vi "Clear All.vi"(8 "error in":errorcluster, 11 "MLTFNC in":refnum<class "MLTFNC.lvclass">) -> (0 "error out":errorcluster, 3 "MLTFNC out":refnum<class "MLTFNC.lvclass">)   [LabVIEW 2019, in "MLTFNC.lvlib" / "MLTFNC.lvclass"]
uses:
  Library/MLTFNC.lvclass
  C:/Users/Public/Documents/Development/builds/Instruments/Instruments.lvlibp/Library/Instruments.lvclass
  Library/MLTFNC.lvclass/MLTFNC.ctl
  builds/Instruments/Instruments.lvlibp/Private/Polymorphic/Special/Event from String.vi
  builds/Instruments/Instruments.lvlibp/Accessors/Command with Logging.vi
  builds/Instruments/Instruments.lvlibp/Library/Instruments.lvclass
  builds/Instruments/Instruments.lvlibp
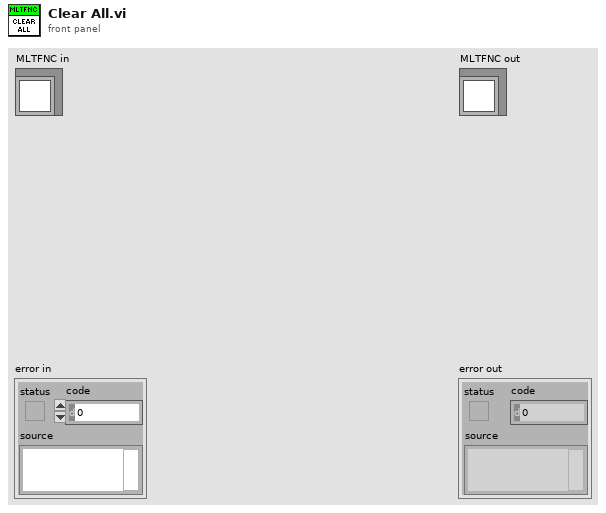
[diagram p1: front panel]
types:
  T1 = cluster{"Timestamp":timestamp, "Description":string, "Data":string}
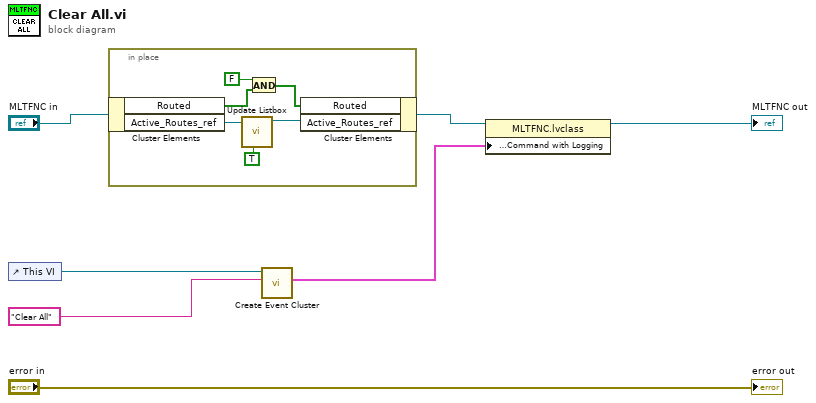
[diagram p0: block diagram]
diagram:
  n1 = control-ref of="This VI"() -> (w3:refnum<vi>)
  n2 = in-place {
    n3 = in-place-cluster #1("MLTFNC in") -> ("Routed"=w10:bool[], "Active_Routes_ref"=w13:refnum<vi>)
    n4 = call "Update Listbox.vi"("Clear"=TRUE, "referencein"=w13) -> ("reference out"=w12:refnum<vi>)  [unwired: 9 in]
    n5 = And(x=FALSE, y=w10) -> (x .and. y?=w8:bool[])
    n6 = in-place-cluster #1("Routed"=w8, "Active_Routes_ref"=w12) -> (w6:refnum<class "MLTFNC.lvclass">)
  }
  n7 = call-poly "Create Event Cluster.vi"("Value"="Clear All", "VI Refnum"=w3) -> ("Event Data"=w2:T1)  [unwired: 9 in]
  n8 = property class="MLTFNC.lvclass"(reference=w6, "Accessors:Logging:Command with Logging"=w2) -> (reference out=→"MLTFNC out":refnum<class "MLTFNC.lvclass">)  [unwired: 1 in, 1 out]
  "error out" <- "error in"
